vi "mqttCmdAcknowledge.vi"(0 "mqttConnect in":refnum<class "mqttCmdConnect.lvclass">, 11 "error in (no error)":errorcluster) -> (4 "mqttConnect out":refnum<class "mqttCmdConnect.lvclass">, 8 "notification":T1, 15 "error out":errorcluster)   [LabVIEW 2013, in "mqttCmdConnect.lvclass"]
uses:
  mqttCmdConnect.lvclass
  mqttTypedef/mqttMessageType.ctl
  mqttTypedef/mqttQOSlevel.ctl
  mqttTypedef/mqttFixedHeaderResponse.ctl
  mqttTypedef/mqttRXdataCluster.ctl
  mqttTypedef/mqttConnectionStatus.ctl
  mqttCmd.lvclass
panel:
  out "payload (HEX)":u8[](array[numeric]) format="%02x"
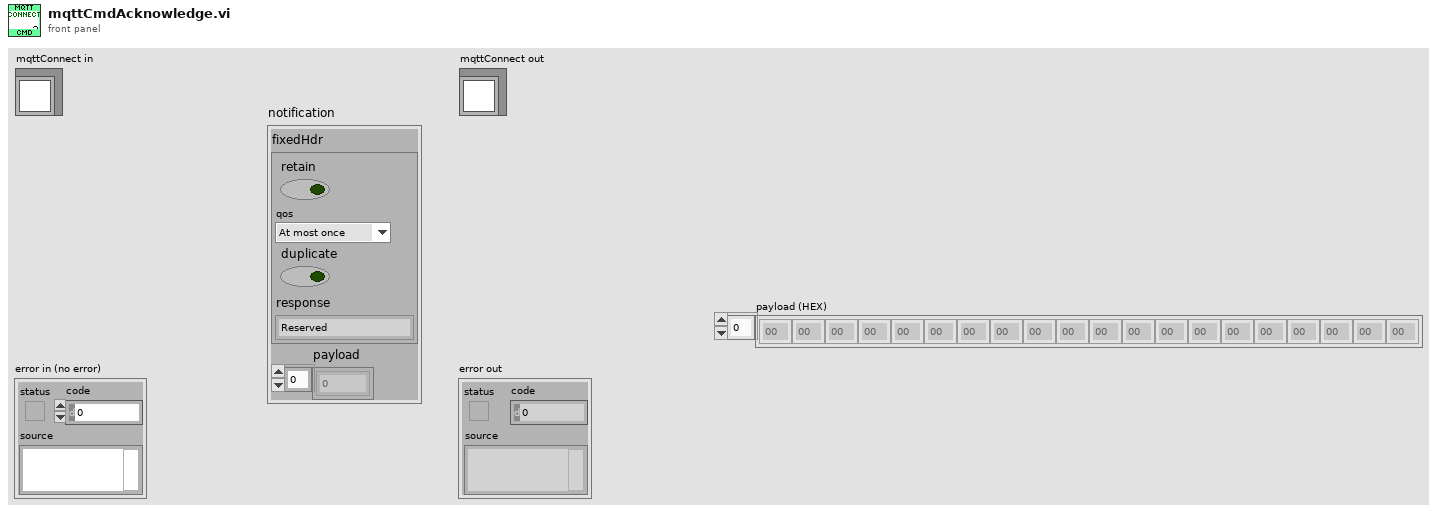
[diagram p1: front panel]
types:
  T1 = typedef "mqttRXdataCluster.ctl" = cluster{"fixedHdr":T2, "payload":u8[]}
  T2 = typedef "mqttFixedHeaderResponse.ctl" = cluster{"retain":bool, "qos":T3, "duplicate":bool, "response":T4}
  T3 = typedef "mqttQOSlevel.ctl" = enum8{"At most once", "At least once", "Exactly once", "Reserved"}
  T4 = typedef "mqttMessageType.ctl" = enum32{"Reserved", "CONNECT", "CONNACK", "PUBLISH", "PUBACK", "PUBREC", "PUBREL", "PUBCOMP", "SUBSCRIBE", "SUBACK", "UNSUBSCRIBE", "UNSUBACK", "PINGREQ", "PINGRESP", "DISCONNECT", "Reserved2"}
  T5 = typedef "mqttConnectionStatus.ctl" = enum16{"Connection accepted", "Connection refused: unacceptable protocol version", "Connection refused: identifier rejected", "Connection refused: Server unavailable", "Connection refused: bad user name or password", "Connection refused: not authorized"}
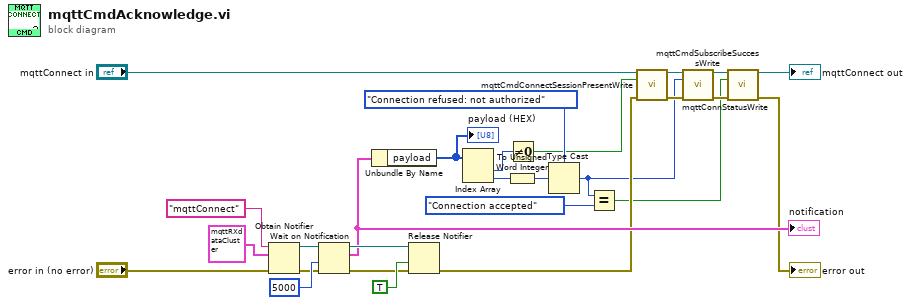
[diagram p0: block diagram]
diagram:
  n1 = Obtain Notifier(name (unnamed)="mqttConnect", notification data type=T1 {"fixedHdr"={"retain"=FALSE, "qos"=enum."At most once", "duplicate"=FALSE, "response"=enum."Reserved"}, "payload"=[]} ("output cluster"), error in (no error)="error in (no error)") -> (notifier out=w23:refnum<notifier>, error out=w22:errorcluster)  [unwired: 1 in, 1 out]
  n2 = Wait on Notification(notifier=w23, timeout in ms (-1)=5000, error in (no error)=w22) -> (notifier out=w26:refnum<notifier>, notification=w14:T1, error out=w25:errorcluster)  [unwired: 1 in, 1 out]
  "notification" <- w14
  n3 = Unbundle By Name(w14) -> ("payload"=w13:u8[])
  "payload (HEX)" <- w13
  n4 = Release Notifier(notifier=w26, force destroy? (F)=TRUE, error in (no error)=w25) -> (error out=w9:errorcluster)  [unwired: 2 out]
  n5 = Index Array(array=w13) -> (element #1=w18:u8, element #2=w16:u8)  [unwired: 2 in]
  n6 = To Unsigned Word Integer(number=w16) -> (unsigned 16bit integer=w15:u16)
  n7 = Not Equal To 0?(x=w18) -> (x != 0?=w12:bool)
  n8 = Type Cast(type=mqttConnectionStatus."Connection refused: not authorized" ("connStatus"), x=w15) -> (*(type *) &x=w2:T5)
  n9 = Equal?(x=w2, y=mqttConnectionStatus."Connection accepted") -> (x = y?=w1:bool)
  n10 = call "mqttCmdConnectSessionPresentWrite.vi"("mqttConnect in"="mqttConnect in", "sessionPresent"=w12, "error in (no error)"=w9) -> ("mqttConnect out"=w10:refnum<class "mqttCmdConnect.lvclass">, "error out"=w8:errorcluster)  [unwired: 11 in]
  n11 = call "mqttConnStatusWrite.vi"("mqttConnect in"=w10, "connStatus"=w2, "error in (no error)"=w8) -> ("mqttConnect out"=w7:refnum<class "mqttCmdConnect.lvclass">, "error out"=w4:errorcluster)  [unwired: 11 in]
  n12 = call "mqttCmdSubscribeSuccessWrite.vi"("mqttBrokerCommand in"=w7, "success"=w1, "error in (no error)"=w4) -> ("mqttBrokerCommand out"=→"mqttConnect out":refnum<class "mqttCmdConnect.lvclass">, "error out"=→"error out":errorcluster)  [unwired: 11 in]
